vi "get inventory from robot.vi"(8 "error in (no error)":errorcluster, 10 "Device selection":refnum<vi>) -> (0 "error out":errorcluster, 3 "Inventory":T1)   [LabVIEW 2016]
uses:
  inventory type def.ctl
  Communication Global variables.vi
  <vilib>/addons/_JKI.lib/REST Client/classes/REST Client/REST Client.lvclass
  <vilib>/addons/_JKI.lib/Serialization/JSON/JKI JSON Serialization.lvlib
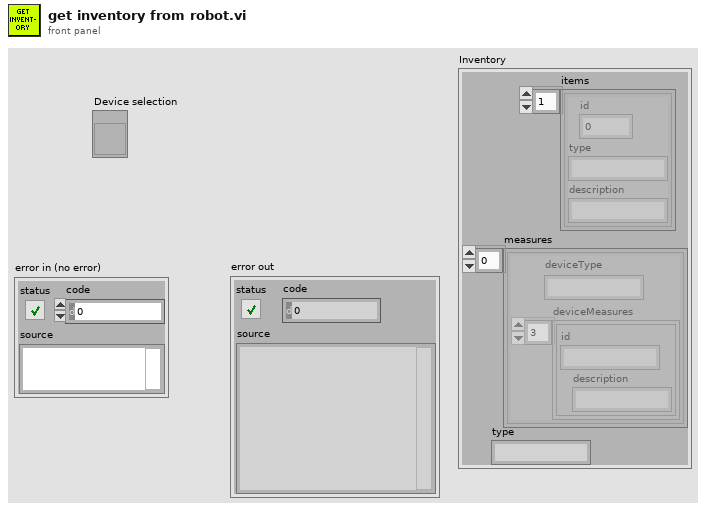
[diagram p1: front panel]
types:
  T1 = typedef "inventory type def.ctl" = cluster{"items":cluster{"id":u8, "type":string, "description":string}[], "measures":cluster{"deviceType":string, "deviceMeasures":cluster{"id":string, "description":string}[]}[], "type":string}
  T2 = cluster{"id":u8, "type":string, "description":string}[]
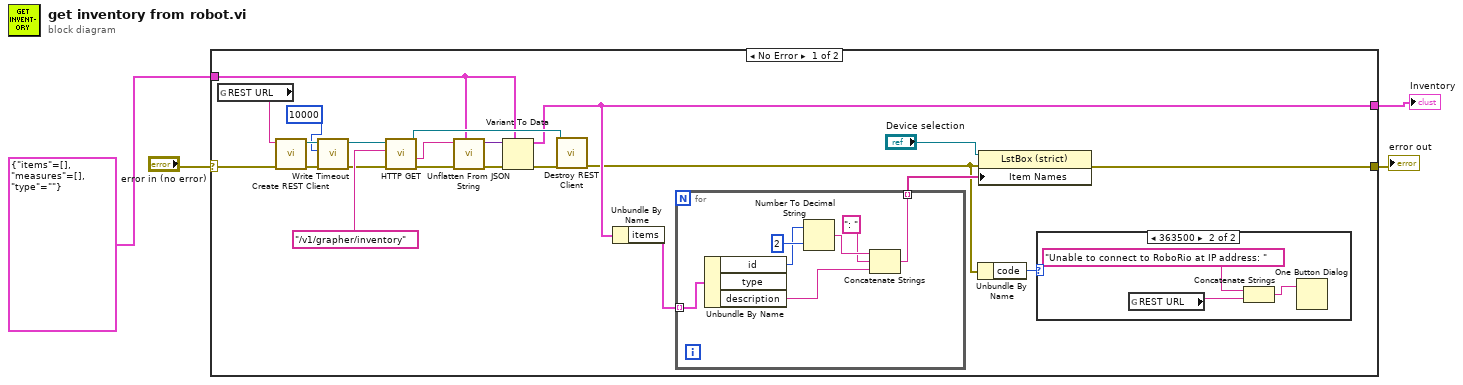
[diagram p0: block diagram]
diagram:
  n1 = case shown="No Error" "error in (no error)" {
    selector: "error in (no error)" -> [w26 w38]
    tunnel: [w20 w38] -> w3
    tunnel: T1 {"items"=[], "measures"=[], "type"=""} -> [w18 w37]
    tunnel: [w22 w37] -> w1
    frame No Error {
      n2 = global read "Communication Global variables.vi" "REST URL"() -> (w14:string)
      n3 = call <vilib>:"Create REST Client.vi"("error in (no error)"=w26, "Base URL"=w14) -> ("error out"=w11:errorcluster, "REST Client out"=w8:refnum<class "REST Client.lvclass">)  [unwired: 8 in]
      n4 = call-dynamic "Write Timeout.vi"("error in (no error)"=w11, "Timeout"=10000, "REST Client in"=w8) -> ("error out"=w10:errorcluster, "REST Client out"=w9:refnum<class "REST Client.lvclass">)  [unwired: 7 in]
      n5 = call-dynamic "HTTP GET.vi"("error in (no error)"=w10, "Path"="/v1/grapher/inventory", "REST Client in"=w9) -> ("error out"=w17:errorcluster, "Response body"=w15:string, "REST Client out"=w24:refnum<class "REST Client.lvclass">)  [unwired: 3 in, 3 out]
      n6 = call <vilib>:"Unflatten From JSON String.vi"("Type and Defaults"=w18, "error in (no error)"=w17, "JSON String"=w15) -> ("error out"=w16:errorcluster, "Variant"=w19:variant)  [unwired: 7 in]
      n7 = Variant To Data(error in=w16, type=w18, Variant=w19) -> (data=w22:T1, error out=w23:errorcluster)
      n8 = call-dynamic "Destroy REST Client.vi"("error in (no error)"=w23, "REST Client in"=w24) -> ("error out"=w6:errorcluster)  [unwired: 9 in]
      n9 = Unbundle By Name(w22) -> ("items"=w21:T2)
      n10 = for {
        tunnel: w21 -> [w36] mode=indexing
        tunnel: [w33] -> w12 mode=indexing
        n11 = Unbundle By Name(w36) -> ("id"=w32:u8, "description"=w35:string)  [unwired: 1 out]
        n12 = Number To Decimal String(number=w32, width (-)=i16 2) -> (decimal integer string=w31:string)
        n13 = Concatenate Strings(w31, ": " ("string"), w35) -> (w33:string)
      }
      n14 = Unbundle By Name(w6) -> ("code"=w5:i32)
      n15 = property class="LstBox (strict)"(reference="Device selection", error in=w6, "Item Names"=w12) -> (error out=w20:errorcluster)  [unwired: 1 out]
      n16 = case shown="363500" w5 {
        frame 0, Default {
        }
        frame 363500 {
          n17 = global read "Communication Global variables.vi" "REST URL"() -> (w29:string)
          n18 = Concatenate Strings("Unable to connect to RoboRio at IP address: " ("message"), w29) -> (w28:string)
          n19 = One Button Dialog(message=w28) -> ()  [unwired: 1 in, 1 out]
        }
      }
    }
    frame Error {
    }
  }
  "error out" <- w3
  "Inventory" <- w1
